vi "Calculate-Cycle time-Higher function.vi"() -> (3 "Cycle Time (s)":dbl)   [LabVIEW 2013]
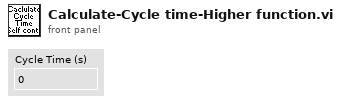
[diagram p1: front panel]
types:
  T1 = typedef "Header parameters cluster-Zstack.ctl" = cluster{"Number of POI":u16, "Number of Miniscans":u16, "Number of Trials":u16, "Number of Cycles ":u16, "# Averaged Frames":u16, "Laser power (%)":u8, "Pockels":dbl, "Acquisition Length (sec)":dbl, "Fill time (us)":dbl, "DwellTime (us)":dbl, "Miniscan Dwell time per pixel (us)":dbl, "PMT 1":dbl, "PMT 2":dbl, "Back Apperture":dbl, "Zoom":dbl, "Number of Pixels in Miniscan":u16, "Frame Size":T2, "Field of View":dbl, "X centre":dbl, "Y centre":dbl, "AOL Z":dbl}
  T2 = typedef "Frame Size.ctl" = u16
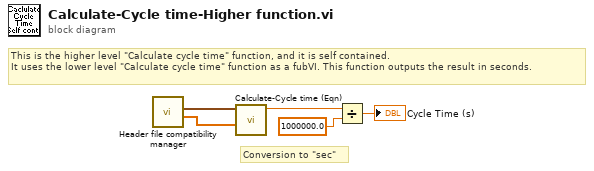
[diagram p0: block diagram]
diagram:
  # "Conversion to \"sec\""
  # "This is the higher level \"Calculate cycle time\" function, and it is self contained.\nIt uses the lower level \"Calculate cycle time\" function as a fubVI. This function outputs the result in seconds."
  n1 = call "Header file compatibility manager.vi"() -> ("[ROI Time (us)]"=w2:dbl[], "Z-Stack Header data"=w1:T1)  [unwired: 8 in, 2 out]
  n2 = call "Calculate-Cycle time (Eqn).vi"("[ROI Time (us)]"=w2, "Header data"=w1) -> ("Cycle Time (us)"=w4:dbl)  [unwired: 9 in]
  n3 = Divide(x=w4, y=1000000.0) -> (x/y=→"Cycle Time (s)":dbl)
